vi "ICNC Push Pulses Data.vi"(7 "BufferRequired":u32, 8 "error in (no error)":errorcluster caption="entrée d'erreur (pas d'erreur)", 9 "Frequency":u32, 10 "nbBytes":i32, 11 "ptBuffer":string) -> (0 "error out":errorcluster caption="sortie d'erreur", 2 "function return":u32, 3 "ptBuffer out":string, 5 "BufferRequired out":u32)   [LabVIEW 2012, in "ICNC2.lvlib"]
doc: "DWORD ICNC_PushPulsesData ( unsigned char *ptBuffer,\n int nbBytes,\n DWORD Frequency,\n DWORD *BufferRequired=NULL);"
uses:
  <userlib>/ICNC/ICNC2.lvlib
  <userlib>/ICNC/ICNC2.dll
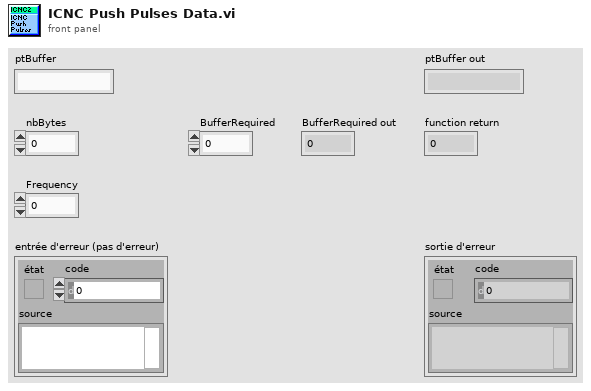
[diagram p1: front panel]
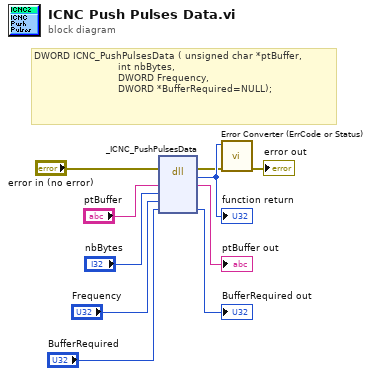
[diagram p0: block diagram]
diagram:
  # "DWORD ICNC_PushPulsesData ( unsigned char *ptBuffer,\n                            int nbBytes,\n                            DWORD Frequency,\n                            DWORD *BufferRequired=NULL);"
  n1 = dll-call lib="C:/Program Files (x86)/National Instruments/LabVIEW 2012/user.lib/ICNC/ICNC2.*" fn="_ICNC_PushPulsesData"(error in="error in (no error)", "ptBuffer"="ptBuffer", "nbBytes"="nbBytes", "Frequency"="Frequency", "BufferRequired"="BufferRequired") -> (error out=w2:errorcluster, w10:u32, "ptBuffer"=→"ptBuffer out":string, "BufferRequired"=→"BufferRequired out":u32)  [unwired: 4 in, 1 out]
  "function return" <- w10
  n2 = call <userlib>:"Error Converter (ErrCode or Status).vi"("error in (no error)"=w2, "error code"=w10) -> ("error out"=→"error out":errorcluster)  [unwired: 9 in]
